vi "Get Common Analog Vars.vi"(1 "All issues in Alm list":bool, 11 "error in (no error)":errorcluster) -> (4 "Catagorised  Stsaus":T1[](array[typedef]), 6 "Values":dbl[](array[numeric]), 8 "Analog Vars":T4[](array[typedef]) {"Value" format="%#.1f"}, 10 "Alarm":bool, 12 "Issue Alarm strings":string[][](array[string]), 13 "Action":T3 items=["No Action", "Turn Off HV"], 14 "Alarms":bool[](array[boolean]), 15 "error out":errorcluster)   [LabVIEW 2011]
uses:
  Action Analog Handler.ctl
  Common/Variable List Common Analog.ctl
  GUI/Analog Var Disp 0 sif.ctl
  GUI/Status indicator Black Small.ctl
  Action List.ctl
  GUI/Status Indikator Helper.ctl
  Catagorised alarm state.ctl
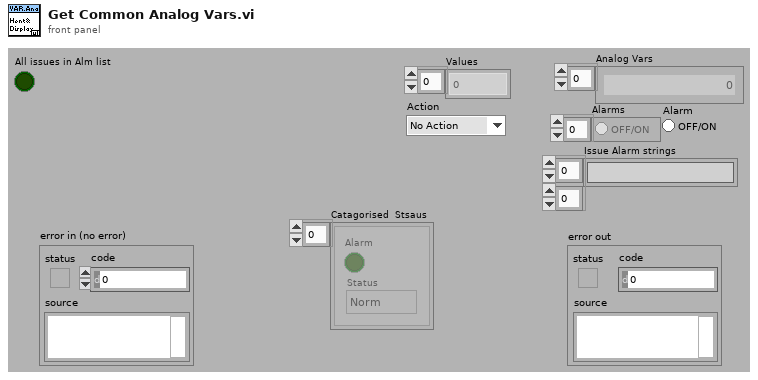
[diagram p1: front panel]
types:
  T1 = typedef "Catagorised alarm state.ctl" = cluster{"Alarm":bool, "Status":T2}
  T2 = typedef "Status Indikator Helper.ctl" = enum16{"Norm", "L", "H", "LL", "HH", "Value", "Technical"}
  T3 = typedef "Action List.ctl" = u16
  T4 = typedef "Analog Var Disp 0 sif.ctl" = cluster{"Value":dbl, "Unit":string, "Status":T5}
  T5 = typedef "Status indicator Black Small.ctl" = u16
  T6 = typedef "Variable List Common Analog.ctl" = enum16{"HVPSU Head Voltage", "HVPSU TS Voltage", "HVPSU Current", "PCP Cable Resistance", "Winch Depth", "Winch Line Speed", "Winch Wire Tension"}
  T7 = typedef "Action Analog Handler.ctl" = enum16{"GET value", "GET Single Frequenzy", "GET All Values", "GET Waveform", "Get Numb Var", "SET Value", "START Buffer", "REG Variable", "BUF size(total antal sekund)", "PULS", "Get a Value at time"}
  T8 = typedef "User Setting Analog Channel Bg.ctl" = cluster{"Scaling":T9, "Limits and responces":T10, "Allow Graph selection by user":bool}
  T9 = typedef "Scaling.ctl" = cluster{"Gain":dbl, "Offset":dbl}
  T10 = typedef "Alarm Setup Analog.ctl" = cluster{"Technical Error(NA)":T11, "LL":T11, "L":T11, "H":T11, "HH":T11, "Limits":T12}
  T11 = typedef "Alarm Responce.ctl" = cluster{"Action":T3, "Alarm":bool}
  T12 = typedef "Limits.ctl" = cluster{"LL":dbl, "L":dbl, "H":dbl, "HH":dbl}
  T13 = typedef "Fixed Analog Channel Definition.ctl" = cluster{"ID":u16, "Name":string, "Unit":string, "Maximum upd":T14, "Comment":string, "Help file Name":string, "Help file Section ":string, "Catagory":T15, "User adjustable Scaling":bool, "Default Scaling":T9, "In use":bool}
  T14 = typedef "Update frequensies.ctl" = enum16{"2 Hz", "1 Hz", "0.1 Hz"}
  T15 = typedef "Channel catagory Enum.ctl" = enum16{"No Catagory", "Power", "Temperature", "Pressure"}
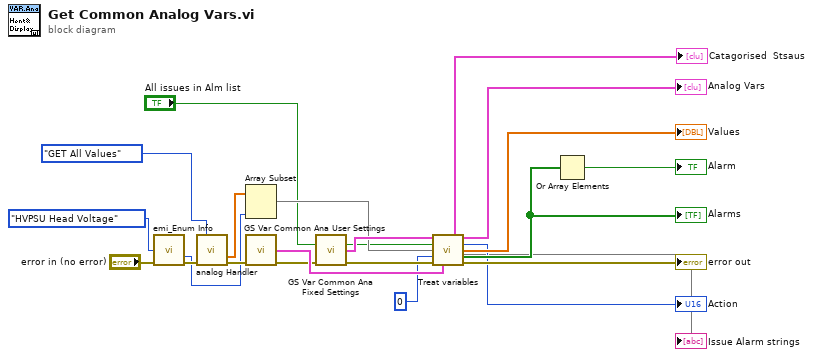
[diagram p0: block diagram]
diagram:
  n1 = call "emi_Enum Info.vi"("Enum"=Variable_List_Common_Analog."HVPSU Head Voltage" ("Action"), "error in (no error)"="error in (no error)") -> ("Numb Elements"=w6:i32, "error out"=w9:errorcluster)  [unwired: 10 in, 2 out]
  n2 = call "analog Handler.vi"("Action"=Action_Analog_Handler."GET All Values" ("Action(GET)"), "error in (no error)"=w9) -> ("Values"=w19:dbl[], "error out"=w8:errorcluster)  [unwired: 8 in, 4 out]
  n3 = Array Subset(array=w19, length=w6) -> (w7:dbl[])  [unwired: 1 in]
  n4 = call "GS Var Common Ana User Settings.vi"("error in (no error)"=w8) -> ("Common Analog var User set out"=w20:T8[], "error out"=w17:errorcluster)  [unwired: 12 in, 1 out]
  n5 = call "GS Var Common Ana Fixed Settings.vi"("error in (no error)"=w17) -> ("Common Analog Var Fixed out"=w21:T13[], "error out"=w22:errorcluster)  [unwired: 12 in, 1 out]
  n6 = call "Treat variables.vi"("Analog Variable info fixed"=w21, "Common alarm handling(F)"="All issues in Alm list", "Analog values"=w7, "Variabel start index"=0, "error In"=w22, "Analog Variable info Settings"=w20) -> ("Catagorised  Stsaus"=→"Catagorised  Stsaus":T1[], "Analog Variable Display"=→"Analog Vars":T4[], "Action"=→"Action":T3, "Analog Values"=→"Values":dbl[], "Alarms"=w15:bool[], 14:→"Issue Alarm strings", "error out"=→"error out":errorcluster)  [unwired: 3 in]
  "Alarms" <- w15
  n7 = Or Array Elements(Boolean array=w15) -> (logical OR=→"Alarm":bool)
